vi "Option Parser.vi"(0 "Tektronix PA1000 in":refnum<class "Tektronix PA1000.lvclass">, 1 "ID":string, 3 "Number of Cards":dbl, 4 "ID cluster.Model":string, 5 "error in (no error)":errorcluster, 7 "Option":string) -> (14 "Tektronix PA1000 out":refnum<class "Tektronix PA1000.lvclass">, 19 "error out":errorcluster)   [LabVIEW 2013, in "Generic Power Analyzer.lvlib" / "Tektronix PA1000.lvlib" / "Tektronix PA1000.lvclass"]
uses:
  Tektronix PA1000.lvclass
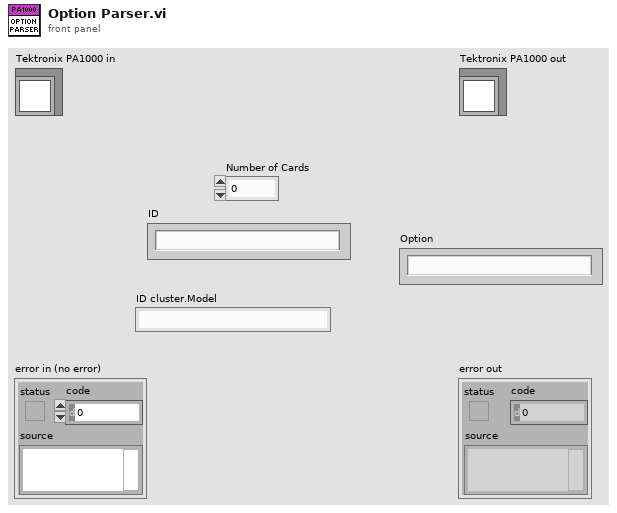
[diagram p1: front panel]
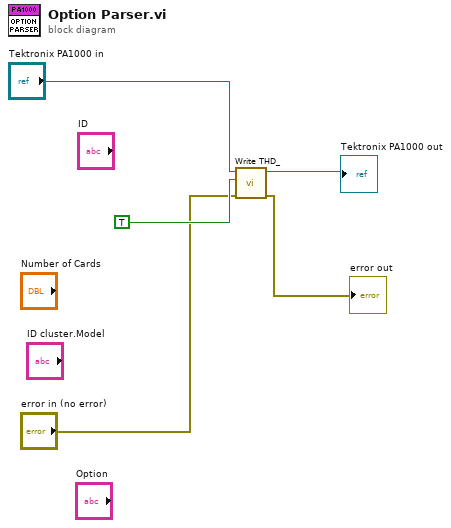
[diagram p0: block diagram]
diagram:
  n1 = call-dynamic "Write THD_.vi"("error in (no error)"="error in (no error)", "THD?"=TRUE, "Generic Power Analyzer in"="Tektronix PA1000 in") -> ("error out"=→"error out":errorcluster, "Generic Power Analyzer out"=→"Tektronix PA1000 out":refnum<class "Tektronix PA1000.lvclass">)  [unwired: 7 in]
